vi "ResetTargets.vi"(8 "error in (no error)":errorcluster, 11 "Bouncer in":refnum<class "Bouncer.lvclass">) -> (0 "error out":errorcluster, 3 "Bouncer out":refnum<class "Bouncer.lvclass">)   [LabVIEW 2019, in "RT_Game.lvlib" / "Bouncer.lvclass"]
uses:
  Bouncer.lvclass
  C:/Users/FreshBob/Dropbox/VIs/myRIO_GameConsole/RT/RT_Game/Game/Game.lvclass
  GridData.ctl
  Bouncer.lvclass/Bouncer.ctl
  BounceTarget/BounceTarget.lvclass
  C:/Users/FreshBob/Dropbox/VIs/myRIO_GameConsole/RT/RT_Game/GameObject/GameObject.lvclass
  GameObject/GameObject.lvclass/GameObject.ctl
  BounceTarget/BounceTarget.lvclass/BounceTarget.ctl
  BounceTarget/Write Position_Tiles.vi
  GameObject/Write size.vi
  GameObject/Write IsActive.vi
  BounceTarget/Write Lives.vi
  GameObject/Write position.vi
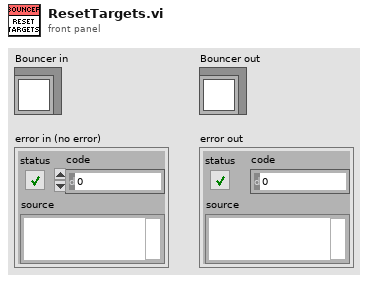
[diagram p1: front panel]
types:
  T1 = typedef "RT_Game.lvlib/Bouncer.lvclass/GridData.ctl" = cluster{"x_count":i8, "y_count":i8, "x_size":i8, "y_size":i8, "x_spacing":i8, "y_spacing":i8, "x_offset":i8, "y_offset":i8}
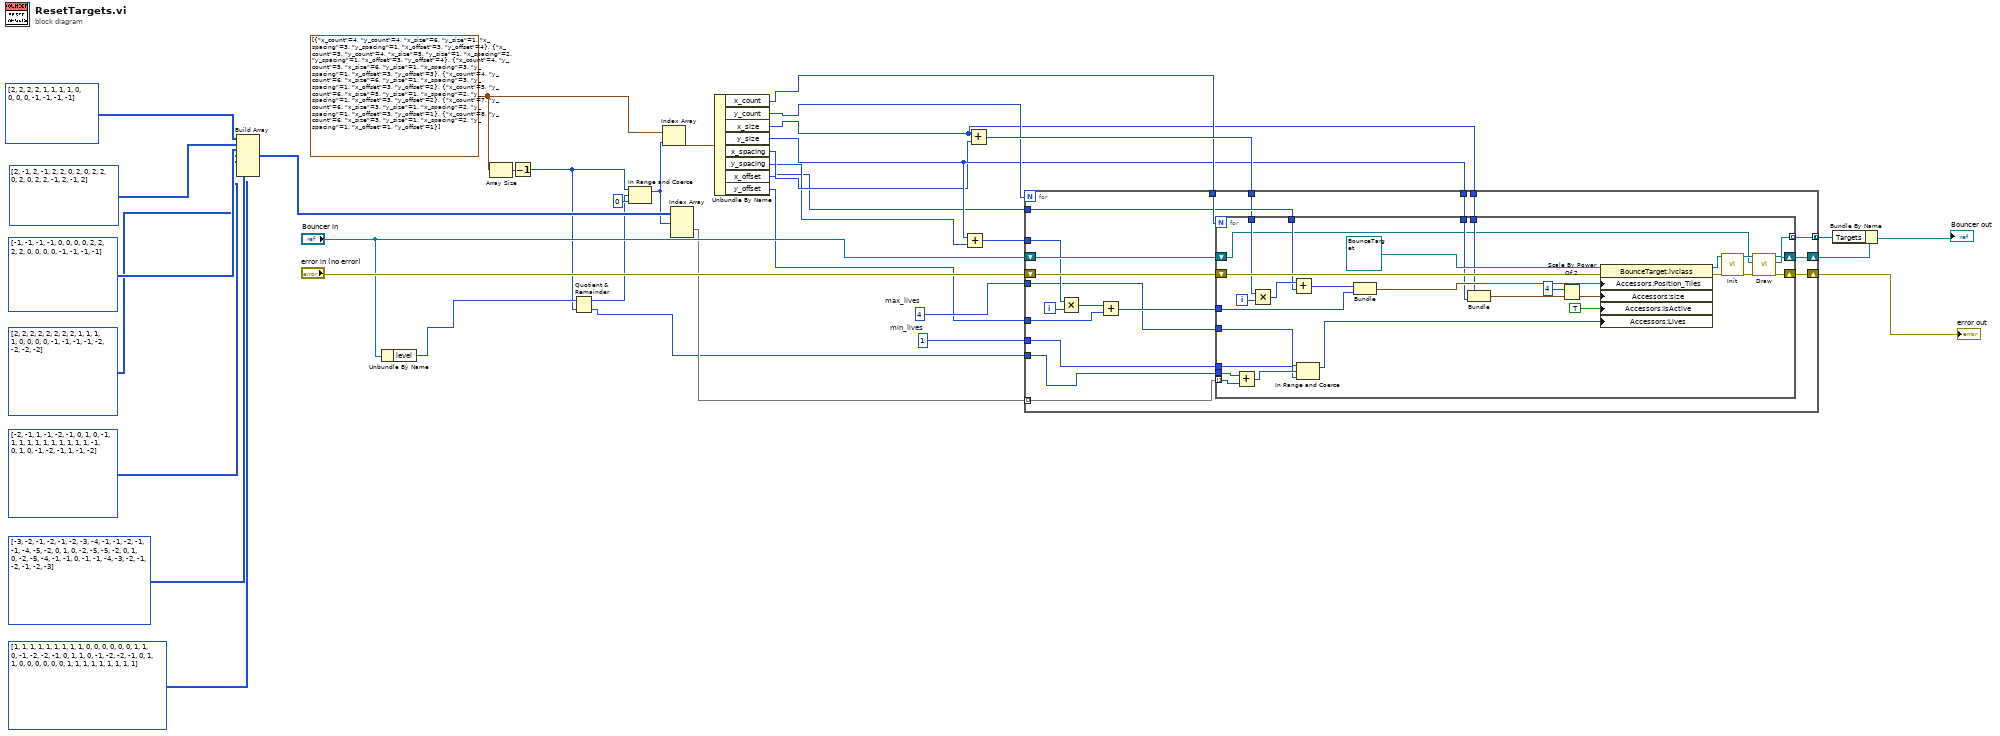
[diagram p0: block diagram]
diagram:
  w20 = T1[] [{"x_count"=4, "y_count"=4, "x_size"=6, "y_size"=1, "x_spacing"=3, "y_spacing"=1, "x_offset"=3, "y_offset"=4}, {"x_count"=5, "y_count"=4, "x_size"=5, "y_size"=1, "x_spacing"=2, "y_spacing"=1, "x_offset"=3, "y_offset"=4}, {"x_count"=4, "y_count"=5, "x_size"=6, "y_size"=1, "x_spacing"=3, "y_spacing"=1, "x_offset"=3, "y_offset"=3}, {"x_count"=4, "y_count"=6, "x_size"=6, "y_size"=1, "x_spacing"=3, "y_spacing"=1, "x_offset"=3, "y_offset"=2}, {"x_count"=5, "y_count"=6, "x_size"=5, "y_size"=1, "x_spacing"=2, "y_spacing"=1, "x_offset"=3, "y_offset"=2}, {"x_count"=7, "y_count"=6, "x_size"=3, "y_size"=1, "x_spacing"=2, "y_spacing"=1, "x_offset"=3, "y_offset"=1}, {"x_count"=8, "y_count"=6, "x_size"=3, "y_size"=1, "x_spacing"=2, "y_spacing"=1, "x_offset"=1, "y_offset"=1}]
  w27 = 4  # max_lives
  w28 = i16 1  # min_lives
  n1 = Build Array(i8[][] [[2, 2, 2, 2], [1, 1, 1, 1], [0, 0, 0, 0], [-1, -1, -1, -1]] ("max_lives"), i8[][] [[2, -1, 2, -1, 2], [2, 0, 2, 0, 2], [2, 0, 2, 0, 2], [2, -1, 2, -1, 2]] ("max_lives"), i8[][] [[-1, -1, -1, -1], [0, 0, 0, 0], [2, 2, 2, 2], [0, 0, 0, 0], [-1, -1, -1, -1]] ("max_lives"), i8[][] [[2, 2, 2, 2], [2, 2, 2, 2], [1, 1, 1, 1], [0, 0, 0, 0], [-1, -1, -1, -1], [-2, -2, -2, -2]] ("max_lives"), i8[][] [[-2, -1, 1, -1, -2], [-1, 0, 1, 0, -1], [1, 1, 1, 1, 1], [1, 1, 1, 1, 1], [-1, 0, 1, 0, -1], [-2, -1, 1, -1, -2]] ("max_lives"), i8[][] [[-3, -2, -1, -2, -1, -2, -3], [-4, -1, -1, -2, -1, -1, -4], [-5, -2, 0, 1, 0, -2, -5], [-5, -2, 0, 1, 0, -2, -5], [-4, -1, -1, 0, -1, -1, -4], [-3, -2, -1, -2, -1, -2, -3]] ("max_lives"), i8[][] [[1, 1, 1, 1, 1, 1, 1, 1], [1, 0, 0, 0, 0, 0, 0, 1], [1, 0, -1, -2, -2, -1, 0, 1], [1, 0, -1, -2, -2, -1, 0, 1], [1, 0, 0, 0, 0, 0, 0, 1], [1, 1, 1, 1, 1, 1, 1, 1]] ("max_lives")) -> (w9:i8[][][])
  n2 = Unbundle By Name("Bouncer in") -> ("level"=w5:i16)
  n3 = Array Size(array=w20) -> (size(s)=w18:i32)
  n4 = Decrement(x=w18) -> (x-1=w3:i32)
  n5 = Quotient & Remainder(x=w5, y=w3) -> (x-y*floor(x/y)=w1:i32, floor(x/y)=w4:i32)
  n6 = In Range and Coerce(upper limit=w3, x=w1, lower limit=0) -> (coerced(x)=w8:i32)  [unwired: 1 out]
  n7 = Index Array(array=w20, index=w8) -> (element=w21:T1)
  n8 = Index Array(array=w9, index (dim 0)=w8) -> (element=w7:i8[][])  [unwired: 2 in]
  n9 = Unbundle By Name(w21) -> ("x_count"=w26:i8, "y_count"=w25:i8, "x_size"=w24:i8, "y_size"=w23:i8, "x_spacing"=w22:i8, "y_spacing"=w17:i8, "x_offset"=w15:i8, "y_offset"=w16:i8)
  n10 = Add(x=w23, y=w17) -> (x+y=w31:i8)
  n11 = Add(x=w24, y=w22) -> (x+y=w30:i8)
  n12 = for {
    N: w25 -> [_]
    shift-right: [w55] -> w32
    shift-left: "error in (no error)" -> [w54]
    shift-right: [w52] -> w33
    shift-left: "Bouncer in" -> [w53]
    tunnel: [w51] -> w34 mode=concatenating
    tunnel: w26 -> [w48]
    tunnel: w31 -> [w47]
    tunnel: w16 -> [w46]
    tunnel: w15 -> [w45]
    tunnel: w30 -> [w44]
    tunnel: w23 -> [w43]
    tunnel: w24 -> [w42]
    tunnel: w4 -> [w39]
    tunnel: w28 -> [w38]
    tunnel: w27 -> [w37]
    tunnel: w7 -> [w40] mode=indexing
    i -> [w41]
    n13 = Multiply(x=w47, y=w41) -> (x*y=w50:i32)
    n14 = Add(x=w50, y=w46) -> (x+y=w49:i32)
    n15 = for {
      N: w48 -> [_]
      shift-right: [w82] -> w55
      shift-left: w54 -> [w81]
      shift-right: [w80] -> w52
      shift-left: w53 -> [w56]
      tunnel: [w79] -> w51 mode=indexing
      tunnel: w49 -> [w72]
      tunnel: w45 -> [w70]
      tunnel: w44 -> [w69]
      tunnel: w43 -> [w66]
      tunnel: w42 -> [w65]
      tunnel: w40 -> [w61] mode=indexing
      tunnel: w39 -> [w62]
      tunnel: w38 -> [w59]
      tunnel: w37 -> [w58]
      i -> [w75]
      n16 = Add(x=w62, y=w61) -> (x+y=w60:i32)
      n17 = Multiply(x=w69, y=w75) -> (x*y=w74:i32)
      n18 = Add(x=w74, y=w70) -> (x+y=w73:i32)
      n19 = In Range and Coerce(upper limit=w58, x=w60, lower limit=w59) -> (coerced(x)=w57:i32)  [unwired: 1 out]
      n20 = Bundle(w73, w72) -> (w71:cluster{i32, i32})  [unwired: 1 in]
      n21 = Bundle("x_size"=w65, "y_size"=w66) -> (w67:cluster{"x_size":i8, "y_size":i8})  [unwired: 1 in]
      n22 = Scale By Power Of 2(n=i16 4, x=w67) -> (x*2^n=w64:cluster{"x_size":i8, "y_size":i8})
      n23 = property class="BounceTarget.lvclass"(reference=refnum<class "BounceTarget.lvclass"> refnum ("RT_Game.lvlib:BounceTarget.lvclass"), error in=w81, "Accessors:Position_Tiles"=w71, "Accessors:size"=w64, "Accessors:IsActive"=TRUE ("IsActive"), "Accessors:Lives"=w57) -> (reference out=w76:refnum<class "BounceTarget.lvclass">, error out=w78:errorcluster)
      n24 = call-dynamic "Init.vi"("error in (no error)"=w78, "BounceTarget in"=w76) -> ("error out"=w84:errorcluster, "BounceTarget out"=w83:refnum<class "BounceTarget.lvclass">)  [unwired: 8 in]
      n25 = call "Draw.vi"("error in (no error)"=w84, "RT_Game.lvlib:Game.lvclass"=w56, "BounceTarget in"=w83) -> ("error out"=w82:errorcluster, "RT_Game.lvlib:Game.lvclass 2"=w80:refnum<class "Bouncer.lvclass">, "BounceTarget out"=w79:refnum<class "BounceTarget.lvclass">)  [unwired: 6 in]
    }
  }
  "error out" <- w32
  n26 = Bundle By Name(cluster=w33, "Targets"=w34) -> (→"Bouncer out":refnum<class "Bouncer.lvclass">)
